vi "MC AO Out Only Engine.vi"(0 "Unique Notifier Name":string="Not a Name", 11 "AO Channel":string[](array[string])) -> ()   [LabVIEW 2020]
uses:
  External Power Control Type Defs/External Power Notifier Type.ctl
  External Power Control Type Defs/External Power Actions.ctl
  <vilib>/ULx/Create Channel.llb/ULx Create Channel (AO-Voltage-Basic).vi
  <vilib>/ULx/Write.llb/ULx Write (Analog 1D DBL 1Chan 1Samp).vi
panel:
  in  "Power (%)":dbl
  in  "Quit":bool
  in  "Line On Off":bool
  # "Array Elements must be:\n\n1) AO Channel (e.g. Dev0/ao0)"
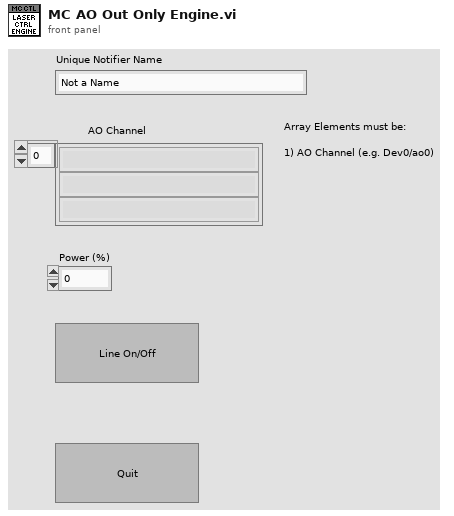
[diagram p1: front panel]
types:
  T1 = typedef "External Power Notifier Type.ctl" = cluster{"Actions":T2, "Wavelength":string, "Line On/Off":bool, "Power (%)":dbl, "Control Parameters":variant, "Cmd Done?":bool}
  T2 = typedef "External Power Actions.ctl" = enum16{"Line On/Off", "Set Power", "Set Ctrl Parameters", "Quit"}
  T3 = enum32{"Invalid", "Standard", "Closed", "Hidden", "Minimized", "Maximized"}
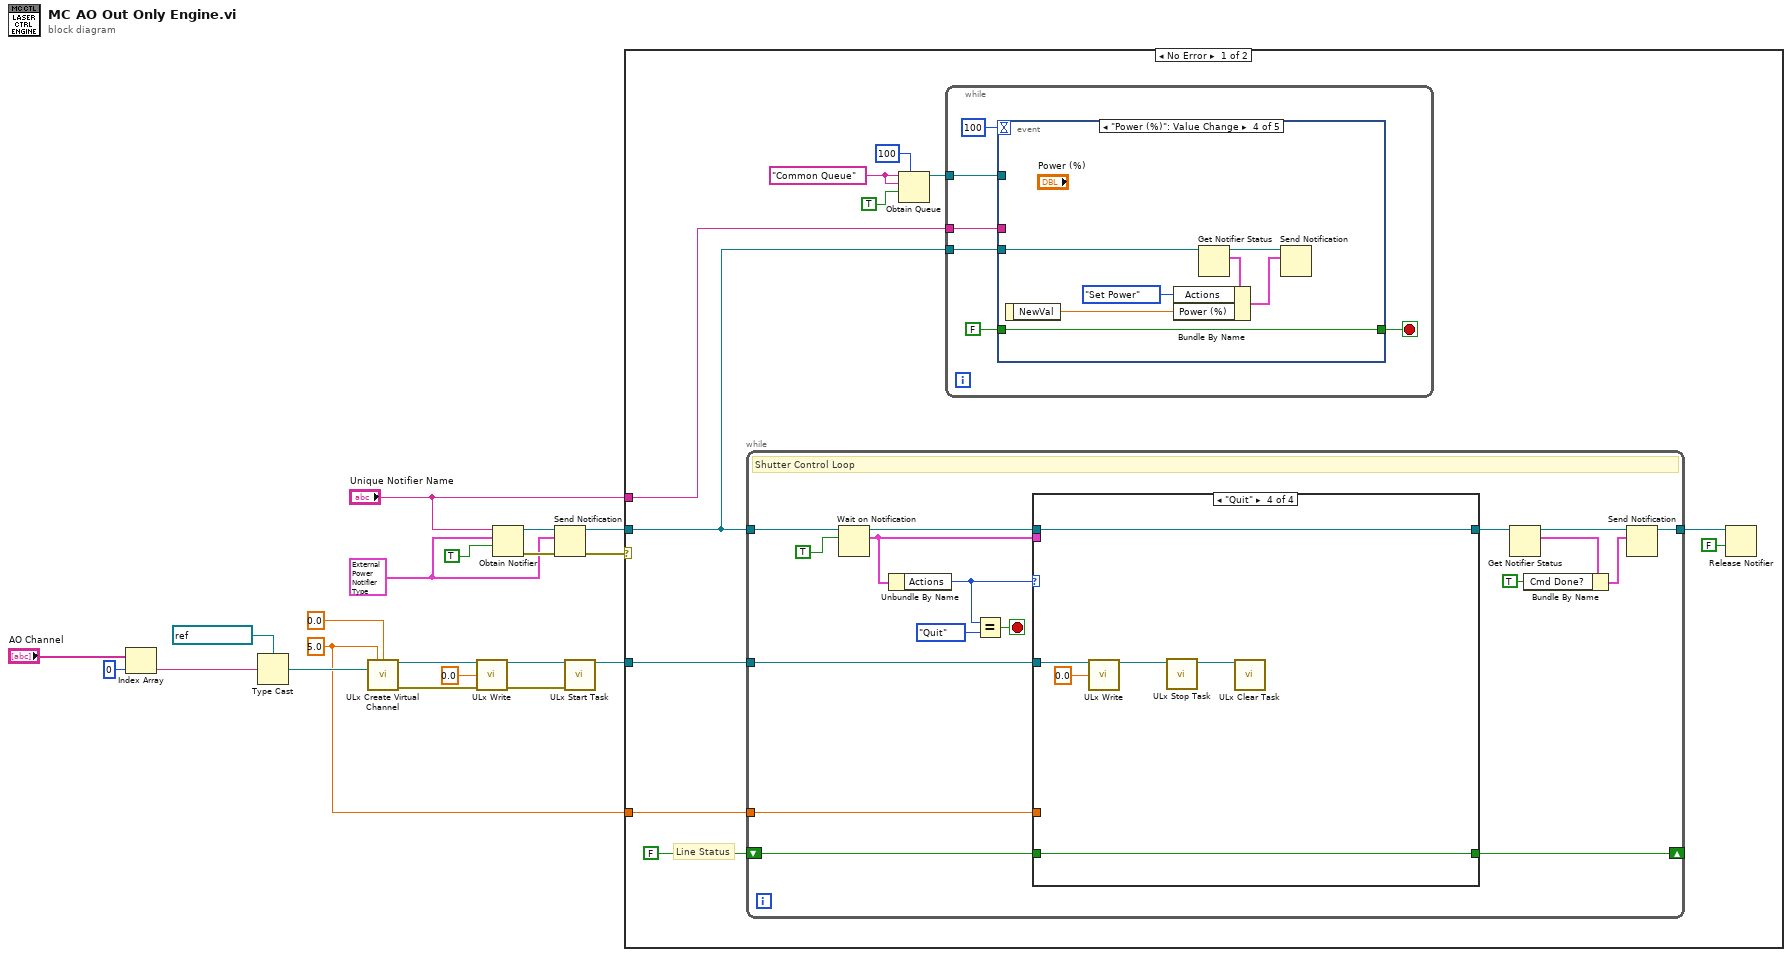
[diagram p0: block diagram]
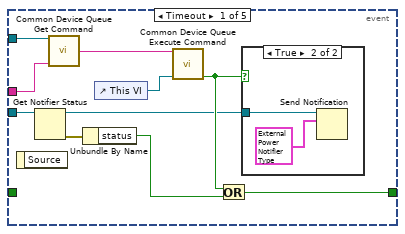
[diagram p2: hidden frame]
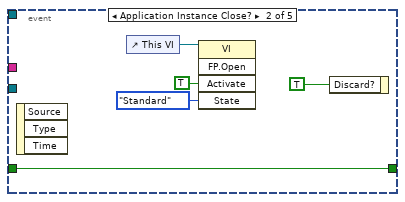
[diagram p4: hidden frame]
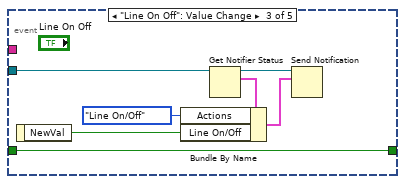
[diagram p5: hidden frame]
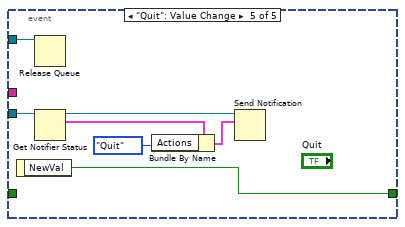
[diagram p6: hidden frame]
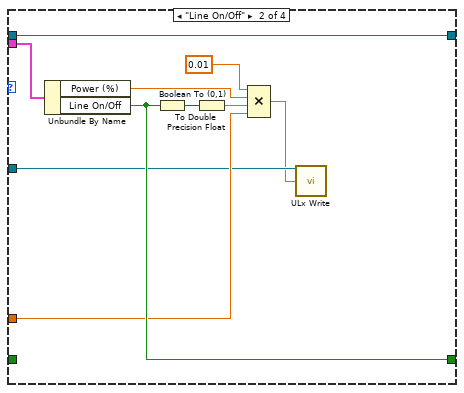
[diagram p8: hidden frame]
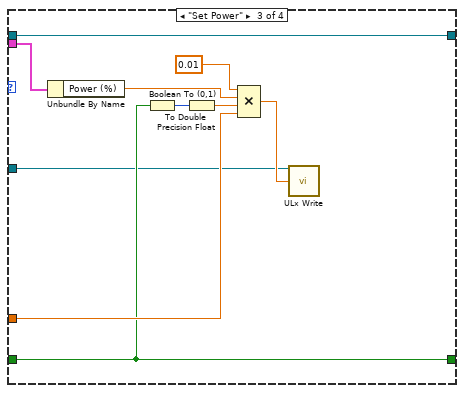
[diagram p9: hidden frame]
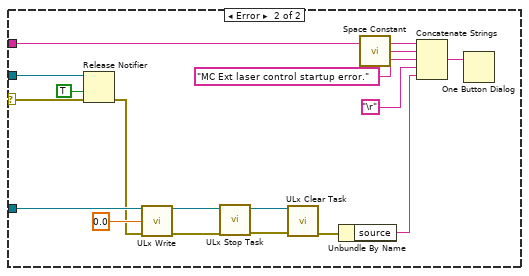
[diagram p10: hidden frame]
diagram:
  w1 = 5.0 ("maximum value")
  w16 = T1 {"Actions"=enum."Set Power", "Wavelength"="", "Line On/Off"=FALSE, "Power (%)"=0.0, "Control Parameters"=variant, "Cmd Done?"=FALSE} ("External Ctrl")
  n1 = Index Array(array="AO Channel", index=0) -> (element=w3:string)
  n2 = Type Cast(type=refnum<k21> "Dev0/Ao0" ("physical channels"), x=w3) -> (*(type *) &x=w9:refnum<k21>)
  n3 = call-poly <vilib>:"ULx Create Virtual Channel.vi"("maximum value"=w1, "minimum value"=0.0, "physical channels"=w9) -> ("task out"=w8:refnum<k24>, "error out"=w7:errorcluster)  [unwired: 11 in]
  n4 = call-poly <vilib>:"ULx Write.vi"("task in"=w8, "data"=0.0, "error in"=w7) -> ("task out"=w5:refnum<k24>, "error out"=w4:errorcluster)  [unwired: 10 in, 1 out]
  n5 = Obtain Notifier(name (unnamed)="Unique Notifier Name", notification data type=w16, create if not found? (T)=TRUE) -> (notifier out=w19:refnum<notifier>, error out=w18:errorcluster)  [unwired: 1 in, 1 out]
  n6 = Send Notification(notification=w16, notifier=w19, error in (no error)=w18) -> (notifier out=w17:refnum<notifier>, error out=w15:errorcluster)
  n7 = call <vilib>:"ULx Start Task.vi"("task in"=w5, "error in"=w4) -> ("task out"=w2:refnum<k24>)  [unwired: 12 in, 1 out]
  n8 = case shown="No Error" w15 {
    selector: w15 -> [_ w135]
    tunnel: w2 -> [w31 w123]
    tunnel: w17 -> [w29 w136]
    tunnel: "Unique Notifier Name" -> [w28 w134]
    tunnel: w1 -> [w22 _]
    frame No Error {
      w27 = "Common Queue" ("Unique Notifier Name")
      # "Line Status"
      n9 = while {
        tunnel: w29 -> [w84]
        tunnel: w31 -> [w90]
        tunnel: [w85] -> w21
        shift-right: [w77] -> _
        shift-left: FALSE -> [w78]
        tunnel: w22 -> [w76]
        stop <- w91 stop-if-true
        # "Shutter Control Loop"
        n10 = Wait on Notification(notifier=w84, ignore previous (F)=TRUE) -> (notifier out=w83:refnum<notifier>, notification=w82:T1)  [unwired: 2 in, 2 out]
        n11 = Unbundle By Name(w82) -> ("Actions"=w81:T2)
        n12 = Equal?(x=w81, y=External_Power_Actions."Quit") -> (x = y?=w91:bool)
        n13 = case shown="\"Quit\"" w81 {
          tunnel: w83 -> [w94 w104 w114 w120]
          tunnel: w90 -> [_ w96 w105 w115]
          tunnel: [w94 w104 w114 w120] -> w88
          tunnel: w82 -> [_ w103 w113 _]
          tunnel: w78 -> [w93 _ w107 w119]
          tunnel: [w93 w101 w107 w119] -> w77
          tunnel: w76 -> [_ w97 w108 _]
          frame Default {
          }
          frame "Line On/Off" {
            n14 = Unbundle By Name(w103) -> ("Power (%)"=w99:dbl, "Line On/Off"=w101:bool)
            n15 = Boolean To (0,1)(Boolean=w101) -> (0, 1=w102:i16)
            n16 = To Double Precision Float(number=w102) -> (double precision float=w100:dbl)
            n17 = Compound Arithmetic op=MULTIPLY(0.01 ("value"), w99, w100, w97) -> (w95:dbl)
            n18 = call-poly <vilib>:"ULx Write.vi"("task in"=w96, "data"=w95) -> ()  [unwired: 11 in, 3 out]
          }
          frame "Set Power" {
            n19 = Unbundle By Name(w113) -> ("Power (%)"=w110:dbl)
            n20 = Boolean To (0,1)(Boolean=w107) -> (0, 1=w112:i16)
            n21 = To Double Precision Float(number=w112) -> (double precision float=w111:dbl)
            n22 = Compound Arithmetic op=MULTIPLY(0.01 ("value"), w110, w111, w108) -> (w106:dbl)
            n23 = call-poly <vilib>:"ULx Write.vi"("task in"=w105, "data"=w106) -> ()  [unwired: 11 in, 3 out]
          }
          frame "Quit" {
            n24 = call-poly <vilib>:"ULx Write.vi"("task in"=w115, "data"=0.0) -> ("task out"=w117:refnum<k24>)  [unwired: 11 in, 2 out]
            n25 = call <vilib>:"ULx Stop Task.vi"("task in"=w117) -> ("task out"=w116:refnum<k24>)  [unwired: 9 in, 1 out]
            n26 = call <vilib>:"ULx Clear Task.vi"("task in"=w116) -> ()  [unwired: 14 in, 1 out]
          }
        }
        n27 = Get Notifier Status(notifier=w88) -> (notifier out=w86:refnum<notifier>, current notification=w89:T1)  [unwired: 1 in, 3 out]
        n28 = Bundle By Name(cluster=w89, "Cmd Done?"=TRUE ("Received?")) -> (w79:T1)
        n29 = Send Notification(notification=w79, notifier=w86) -> (notifier out=w85:refnum<notifier>)  [unwired: 1 in, 1 out]
      }
      n30 = Obtain Queue(max queue size (-1, unlimited)=100, name (unnamed)=w27, element data type=w27, create if not found? (T)=TRUE) -> (queue out=w24:refnum<queue>)  [unwired: 1 in, 2 out]
      n31 = while {
        tunnel: w24 -> [w37]
        tunnel: w29 -> [w34]
        tunnel: w28 -> [w32]
        stop <- w33 stop-if-true
        n32 = event shown="[3] \"Power (%)\": Value Change" {
          selector: _ -> [_ _ _ _ _]
          dyn-events: _ -> [_ _ _ _ _]
          timeout: 100 -> [_ _ _ _ _]
          tunnel: w37 -> [w45 _ _ _ w70]
          tunnel: FALSE -> [_ w54 w57 w64 _]
          tunnel: w34 -> [w47 _ w61 w68 w71]
          tunnel: [w40 w54 w57 w64 w75] -> w33
          tunnel: w32 -> [w44 _ _ _ _]
          event Timeout {
            n33 = event-data() -> ()  [unwired: 1 in, 1 out]
            n34 = Get Notifier Status(notifier=w47) -> (notifier out=w38:refnum<notifier>, error out=w46:errorcluster)  [unwired: 1 in, 3 out]
            n35 = call "Common Device Queue Get Command.vi"("Common Queue"=w45, "Notifier Name"=w44) -> ("Command"=w43:string)  [unwired: 12 in, 1 out]
            n36 = Unbundle By Name(w46) -> ("status"=w41:bool)
            n37 = control-ref of="This VI"() -> (w42:refnum<vi>)
            n38 = call "Common Device Queue Execute Command.vi"("Common Command"=w43, "VI Refnum"=w42) -> ("Quit?"=w39:bool)  [unwired: 12 in, 1 out]
            n39 = Or(x=w39, y=w41) -> (x .or. y?=w40:bool)
            n40 = case shown="True" w39 {
              tunnel: w38 -> [_ w49]
              frame False {
              }
              frame True {
                n41 = Send Notification(notification=T1 {"Actions"=enum."Quit", "Wavelength"="", "Line On/Off"=FALSE, "Power (%)"=0.0, "Control Parameters"=variant, "Cmd Done?"=FALSE} ("External Ctrl"), notifier=w49) -> ()  [unwired: 1 in, 2 out]
              }
            }
          }
          event Application Instance Close? {
            n42 = event-data() -> ()  [unwired: 1 in, 3 out]
            n43 = control-ref of="This VI"() -> (w51:refnum<vi>)
            n44 = invoke class="VI" method="FP.Open"(reference=w51, "Activate"=TRUE ("Activate?"), "State"=T3."Standard") -> ()  [unwired: 2 in, 5 out]
            n45 = event-data("Discard?"=TRUE) -> ()  [unwired: 1 in, 1 out]
          }
          event "Line On Off": Value Change {
            n46 = event-data() -> ("NewVal"=w56:bool)  [unwired: 1 in]
            n47 = Get Notifier Status(notifier=w61) -> (notifier out=w60:refnum<notifier>, current notification=w59:T1)  [unwired: 1 in, 3 out]
            n48 = Bundle By Name(cluster=w59, "Actions"=External_Power_Actions."Line On/Off", "Line On/Off"=w56) -> (w58:T1)
            n49 = Send Notification(notification=w58, notifier=w60) -> ()  [unwired: 1 in, 2 out]
          }
          event "Power (%)": Value Change {
            n50 = event-data() -> ("NewVal"=w63:dbl)  [unwired: 1 in]
            n51 = Get Notifier Status(notifier=w68) -> (notifier out=w67:refnum<notifier>, current notification=w66:T1)  [unwired: 1 in, 3 out]
            n52 = Bundle By Name(cluster=w66, "Actions"=External_Power_Actions."Set Power", "Power (%)"=w63) -> (w65:T1)
            n53 = Send Notification(notification=w65, notifier=w67) -> ()  [unwired: 1 in, 2 out]
          }
          event "Quit": Value Change {
            n54 = event-data() -> ("NewVal"=w75:bool)  [unwired: 1 in]
            n55 = Release Queue(queue=w70) -> ()  [unwired: 2 in, 3 out]
            n56 = Get Notifier Status(notifier=w71) -> (notifier out=w74:refnum<notifier>, current notification=w73:T1)  [unwired: 1 in, 3 out]
            n57 = Bundle By Name(cluster=w73, "Actions"=External_Power_Actions."Quit") -> (w72:T1)
            n58 = Send Notification(notification=w72, notifier=w74) -> ()  [unwired: 1 in, 2 out]
          }
        }
      }
      n59 = Release Notifier(notifier=w21, force destroy? (F)=FALSE) -> ()  [unwired: 1 in, 3 out]
    }
    frame Error {
      n60 = Release Notifier(notifier=w136, force destroy? (F)=TRUE, error in (no error)=w135) -> (error out=w122:errorcluster)  [unwired: 2 out]
      n61 = call-poly <vilib>:"ULx Write.vi"("task in"=w123, "data"=0.0, "error in"=w122) -> ("task out"=w127:refnum<k24>, "error out"=w125:errorcluster)  [unwired: 10 in, 1 out]
      n62 = call <vilib>:"ULx Stop Task.vi"("error in"=w125, "task in"=w127) -> ("error out"=w124:errorcluster, "task out"=w126:refnum<k24>)  [unwired: 8 in]
      n63 = call <vilib>:"ULx Clear Task.vi"("task in"=w126, "error in"=w124) -> ("error out"=w121:errorcluster)  [unwired: 13 in]
      n64 = Unbundle By Name(w121) -> ("source"=w129:string)
      n65 = call <vilib>:"Space Constant.vi"() -> ("String"=w132:string)
      n66 = Concatenate Strings(w134, w132, "MC Ext laser control startup error." ("string"), "\r", w129) -> (w133:string)
      n67 = One Button Dialog(message=w133) -> ()  [unwired: 1 in, 1 out]
    }
  }
